vi "Make DLL Param(Storage Rsp).vi"   [LabVIEW 8.6, in "Keyence LJ-V7000.lvlib"]
uses:
  Keyence LJ-V7000.lvlib
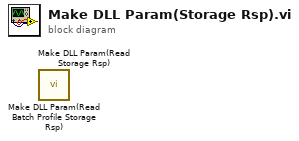
[diagram p0: block diagram]
diagram:
  n1 = call "Make DLL Param(Read Batch Profile Storage Rsp).vi"() -> ()  [unwired: 1 in, 1 out]
  n2 = call "Make DLL Param(Read Storage Rsp).vi"() -> ()  [unwired: 1 in, 1 out]
